vi "_TangoDisplayError.vi"(2 "error in":errorcluster) -> ()   [LabVIEW 2014, in "tango.lvlib"]
uses:
  tango.lvlib
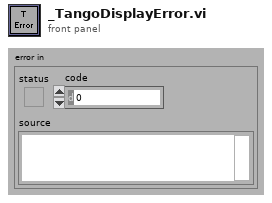
[diagram p1: front panel]
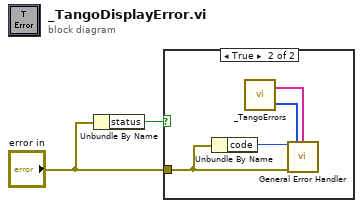
[diagram p0: block diagram]
diagram:
  n1 = Unbundle By Name("error in") -> ("status"=w1:bool)
  n2 = case shown="True" w1 {
    tunnel: "error in" -> [_ w4]
    frame False {
    }
    frame True {
      n3 = Unbundle By Name(w4) -> ("code"=w3:i32)
      n4 = call "_TangoErrors.vi"() -> ("Tango Error codes"=w6:i32[], "Tango error descs"=w5:string[])  [unwired: 2 in]
      n5 = call <vilib>:"General Error Handler.vi"("[error code] (0)"=w3, "[user-defined codes]"=w6, "[user-defined descriptions]"=w5, "error in (no error)"=w4) -> ()  [unwired: 7 in, 5 out]
    }
  }
